vi "Save.vi"() -> (1 "保存数据文件至： 2":path, 2 "数据文件名称： 2":string, 3 "是否取消？":bool)   [LabVIEW 2014]
panel:
  in  "数据文件名称：":string
  in  "取消":bool
  in  "确定":bool
  in  "保存数据文件至：":path
  # "请选择要保存数据文件的文件夹路径。测量结果TXT格式保存。"
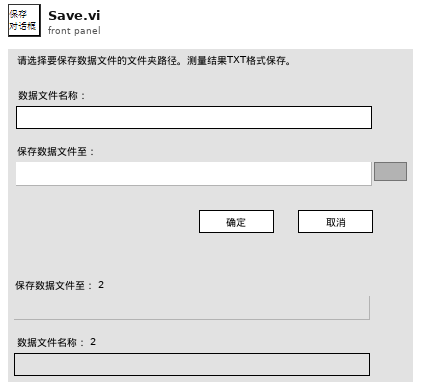
[diagram p1: front panel]
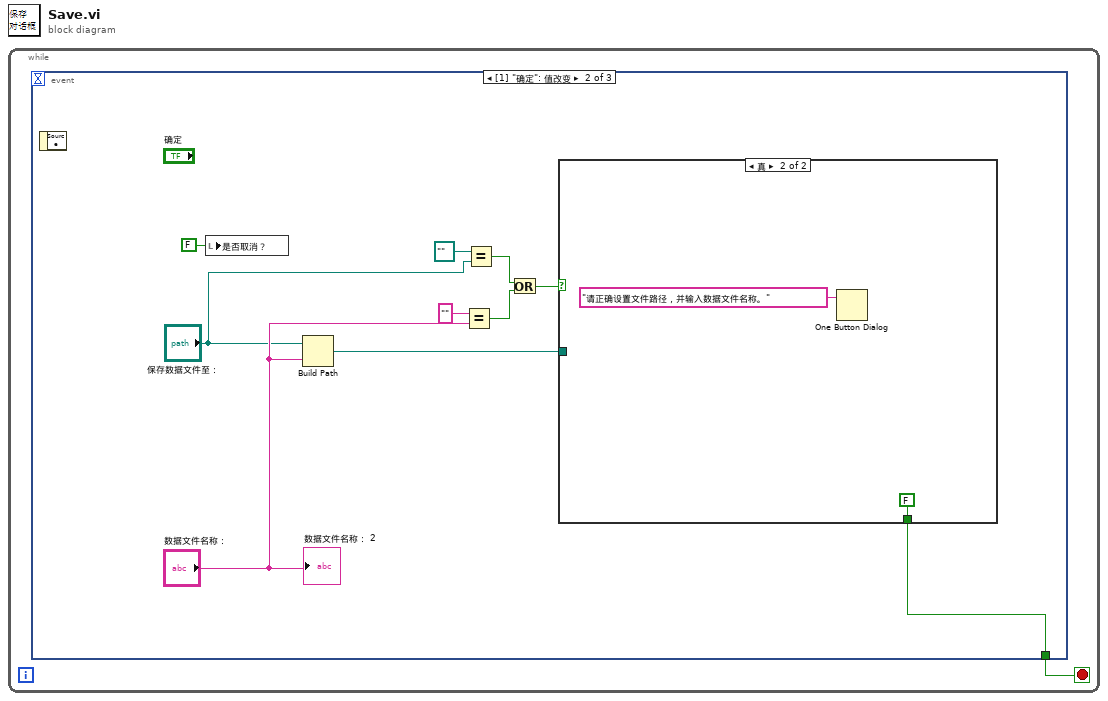
[diagram p0: block diagram]
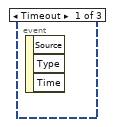
[diagram p2: hidden frame]
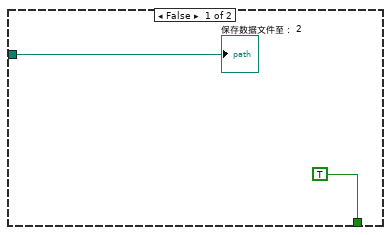
[diagram p3: hidden frame]
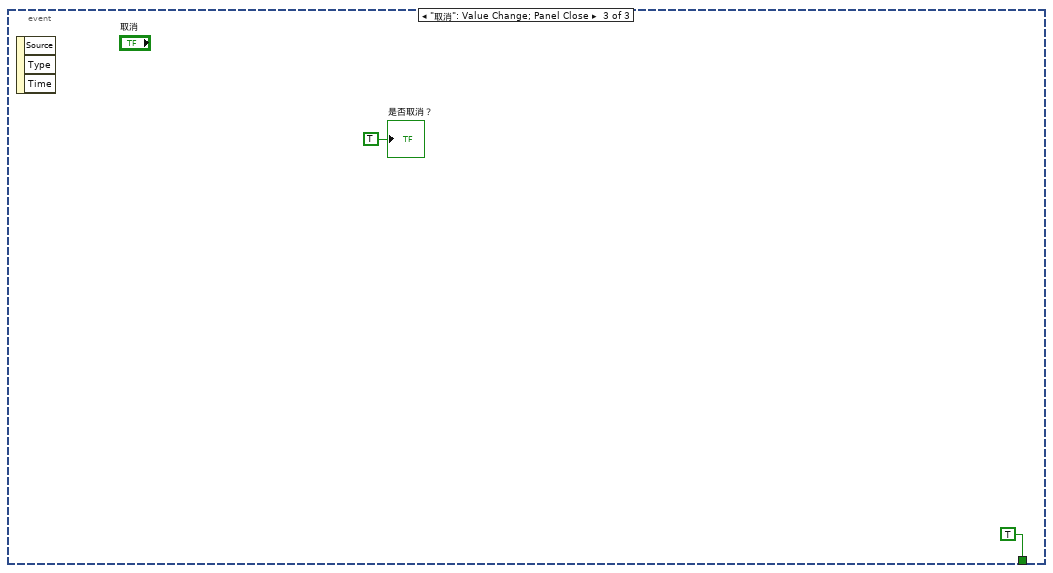
[diagram p4: hidden frame]
diagram:
  n1 = while {
    stop <- w1 stop-if-true
    n2 = event shown="[1] \"确定\": 值改变" {
      selector: _ -> [_ _ _]
      dyn-events: _ -> [_ _ _]
      timeout: _ -> [_ _ _]
      tunnel: [_ w3 TRUE] -> w1
      event Timeout {
        n3 = event-data() -> ()  [unwired: 1 in, 3 out]
      }
      event "确定": Value Change {
        n4 = event-data() -> ()  [unwired: 1 in, 1 out]
        n5 = local write "是否取消？"(FALSE ("是否取消？")) -> ()
        n6 = Build Path(base path="保存数据文件至：", name or relative path="数据文件名称：") -> (appended path=w10:path)
        n7 = Equal?(x="", y="数据文件名称：") -> (x = y?=w6:bool)
        n8 = Equal?(x=path "", y="保存数据文件至：") -> (x = y?=w5:bool)
        n9 = Or(x=w5, y=w6) -> (x .or. y?=w4:bool)
        n10 = case shown="真" w4 {
          tunnel: w10 -> [w13 _]
          tunnel: [TRUE FALSE] -> w3
          frame False {
            "保存数据文件至： 2" <- w13
          }
          frame True {
            n11 = One Button Dialog(message="请正确设置文件路径，并输入数据文件名称。" ("消息")) -> ()  [unwired: 1 in, 1 out]
          }
        }
        "数据文件名称： 2" <- "数据文件名称："
      }
      event "取消": Value Change; Panel Close {
        n12 = event-data() -> ()  [unwired: 1 in, 3 out]
        "是否取消？" <- TRUE ("是否取消？")
      }
    }
  }
